vi "helper_one_button.vi"(1 "message":string, 2 "button_name":string) -> (0 "Boolean":bool)   [LabVIEW 2015, in "lv-dialog.lvlib" / "v1.lvlib"]
uses:
  v1.lvlib
  _controls/configuration.ctl
  _controls/dialog_selection.ctl
  v1.lvclass
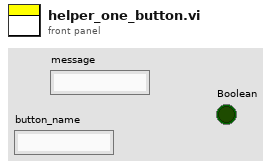
[diagram p1: front panel]
types:
  T1 = typedef "lv-dialog.lvlib/v1.lvlib/dialog_selection.ctl" = enum16{"null", "panel_closed", "button_1", "button_2", "button_3", "cancelled"}
  T2 = typedef "lv-dialog.lvlib/v1.lvlib/configuration.ctl" = cluster{"dialog_text":string, "boolean_text_1":string, "boolean_text_2":string, "boolean_text_3":string, "inner_color":u32, "outer_color":u32, "wait_s":dbl, "error_status":bool, "error_source":string, "error_details":string, "string []":string[], "custom_entry":bool}
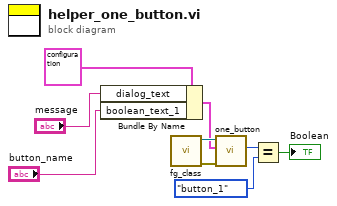
[diagram p0: block diagram]
diagram:
  n1 = Bundle By Name(cluster=T2 {"dialog_text"="", "boolean_text_1"="", "boolean_text_2"="", "boolean_text_3"="", "inner_color"=16711680, "outer_color"=6618880, "wait_s"=nan, "error_status"=FALSE, "error_source"="", "error_details"="", "string []"=[], "custom_entry"=FALSE} ("configuration"), "dialog_text"="message", "boolean_text_1"="button_name") -> (w6:T2)
  n2 = call "fg_class.vi"() -> ("error out"=w8:errorcluster, "class out"=w9:refnum<class "v1.lvclass">)  [unwired: 10 in]
  n3 = call-dynamic "one_button.vi"("error in (no error)"=w8, "configuration"=w6, "v1 in"=w9) -> ("dialog_selection"=w3:T1)  [unwired: 6 in, 2 out]
  n4 = Equal?(x=w3, y=dialog_selection."button_1") -> (x = y?=→"Boolean":bool)
